vi "VISCOSITY.vi"(0 "SPIN (F)":bool, 1 "Zero? (T)":bool=TRUE, 3 "Startup RPM":dbl=6.0, 5 "LogData? (T)":bool=TRUE, 9 "GUID":string, 11 "DataPoints":i32=10, 12 "stabilization (ms)":u32=10000) -> (4 "cP_Array":dbl[](array[numeric]), 6 "TorqueArray":dbl[](array[numeric]), 8 "final_RPM":dbl, 10 "cP_mean":dbl format="%0.2f", 13 "tau_std":dbl format="%0.2f", 14 "ET (s)":dbl, 15 "tau_mean":dbl format="%0.2f")   [LabVIEW 2019]
uses:
  CurrentRevision/5_Controls/Brookfield_type-def.ctl
  <vilib>/Instr/_visa.llb/VISA Flush IO Buffer Mask.ctl
  <vilib>/Utility/error.llb/DialogType.ctl
  <vilib>/Analysis/baseanly.llb/Mean (DBL).vi
  <vilib>/Utility/file.llb/Read Delimited Spreadsheet (DBL).vi
  <vilib>/Analysis/NI_AALBase.lvlib
panel:
  out "READ_COUNT_AT_SPEED":i32
  out "end_time":timestamp
  out "start_time":timestamp
  out "Temp_mean":dbl format="%0.2f"
  out "Coefficient of VariationT":dbl
  out "net tq%":dbl
  out "Desired RPM":dbl
  out "Coefficient of Variation cP":dbl
  out "speed ratio":dbl
  out "cP":dbl
  out "Loop Tracker":T1[](array[typedef])
  out "Zero_write":dbl
  out "Set RPM":dbl
  out "standard dev":dbl format="%0.2f"
  out "Zero_read":dbl
  out "ReconnectAttempts":i32
  out "log_string":string
  out "TempArray":dbl[](array[numeric])
  out "error out":errorcluster
  out "Enum":T1
  out "temp":dbl
  out "abs tq%":dbl
  out "Control Circuitry Enabled":bool
  out "Motor On":bool
  out "Motor Stopped":bool
  out "Auto-zero Complete":bool
  out "Motor Circuit Error":bool
  out "Diagnostics Error":bool
  out "Invalid Command Received":bool
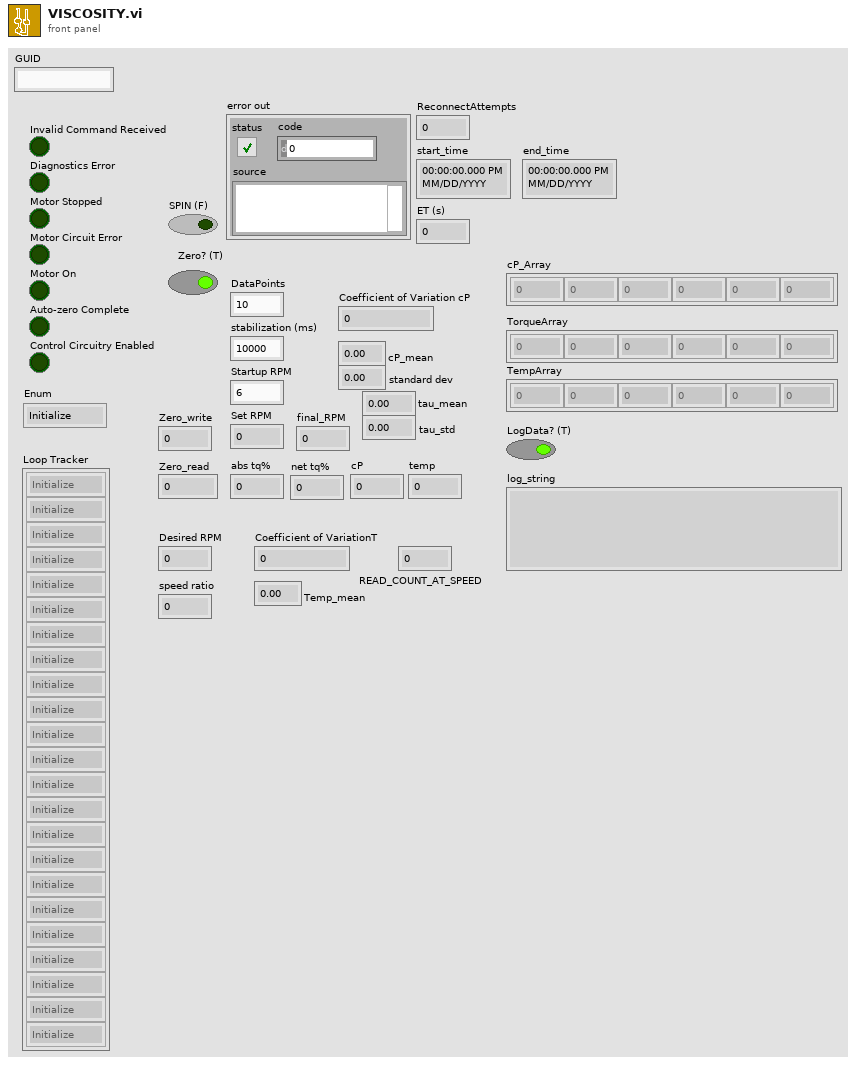
[diagram p1: front panel]
types:
  T1 = typedef "Brookfield_type-def.ctl" = enum16{"Initialize", "Enable", "Ready", "Zero", "Set Speed", "Read", "Stop Motor", "Error", "Disconnect"}
  T2 = enum16{"open", "replace", "create", "open or create", "replace or create", "replace or create with confirmation"}
  T3 = typedef "VISA Flush IO Buffer Mask.ctl" = u16
  T4 = typedef "DialogType.ctl" = u16
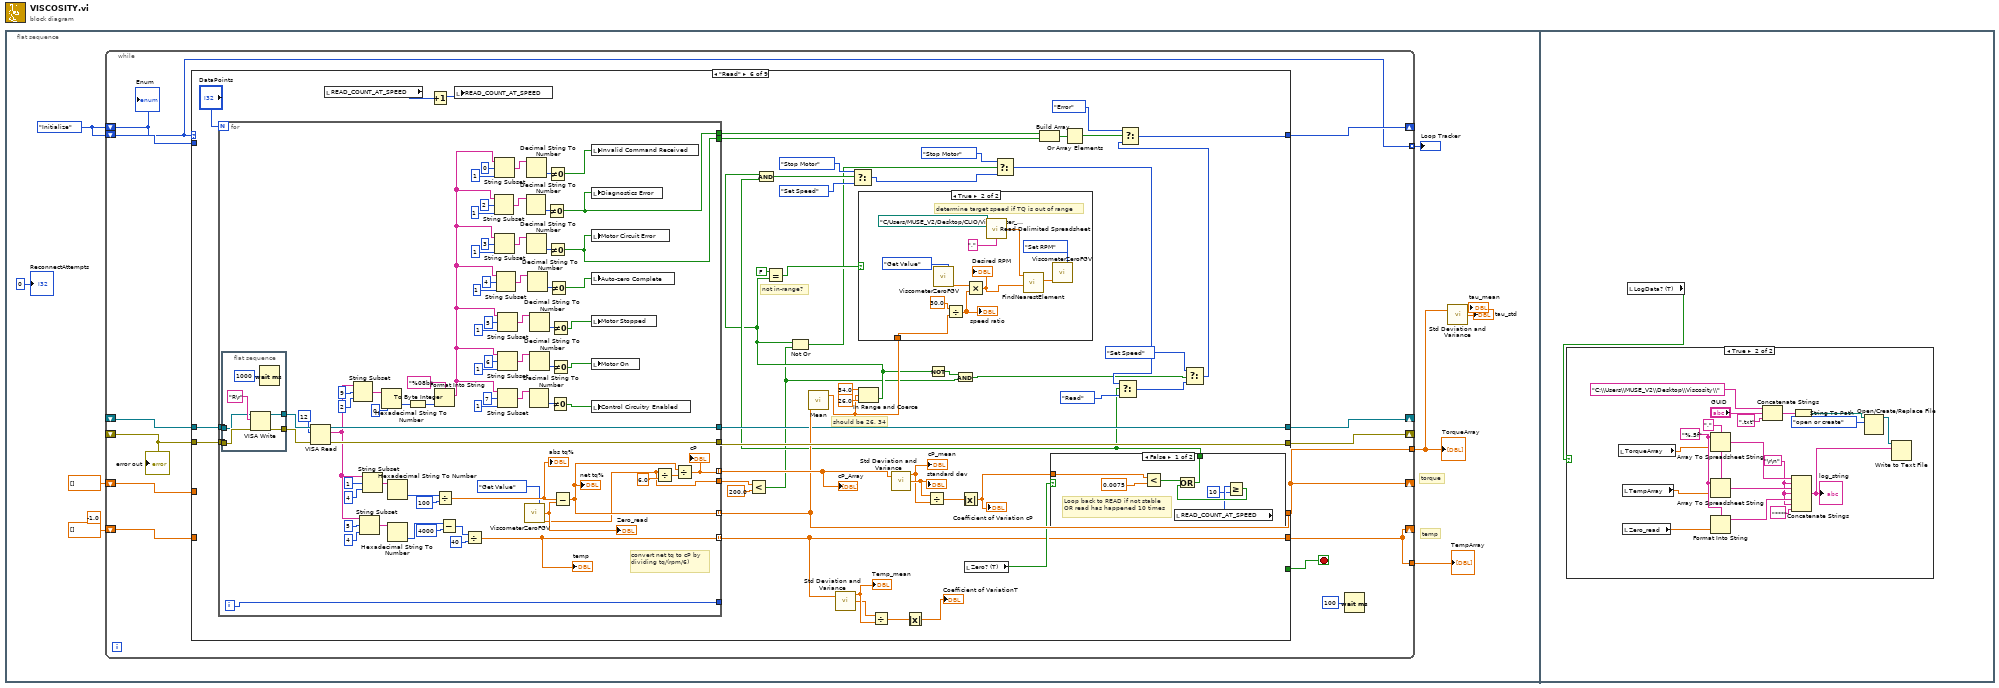
[diagram p0: block diagram]
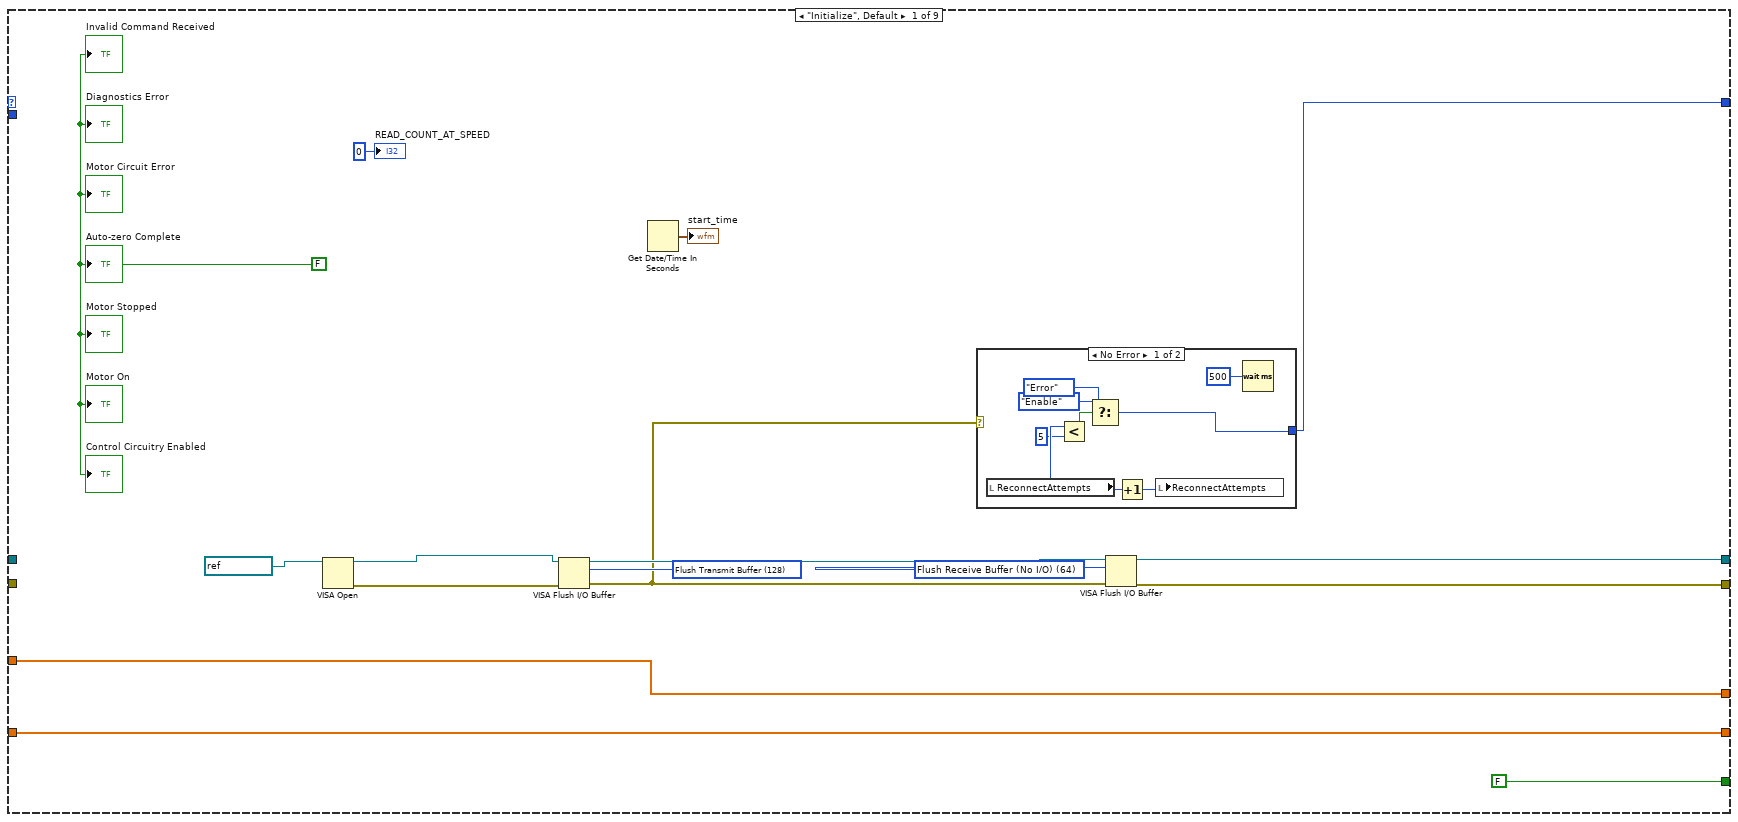
[diagram p2: hidden frame]
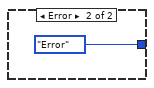
[diagram p3: hidden frame]
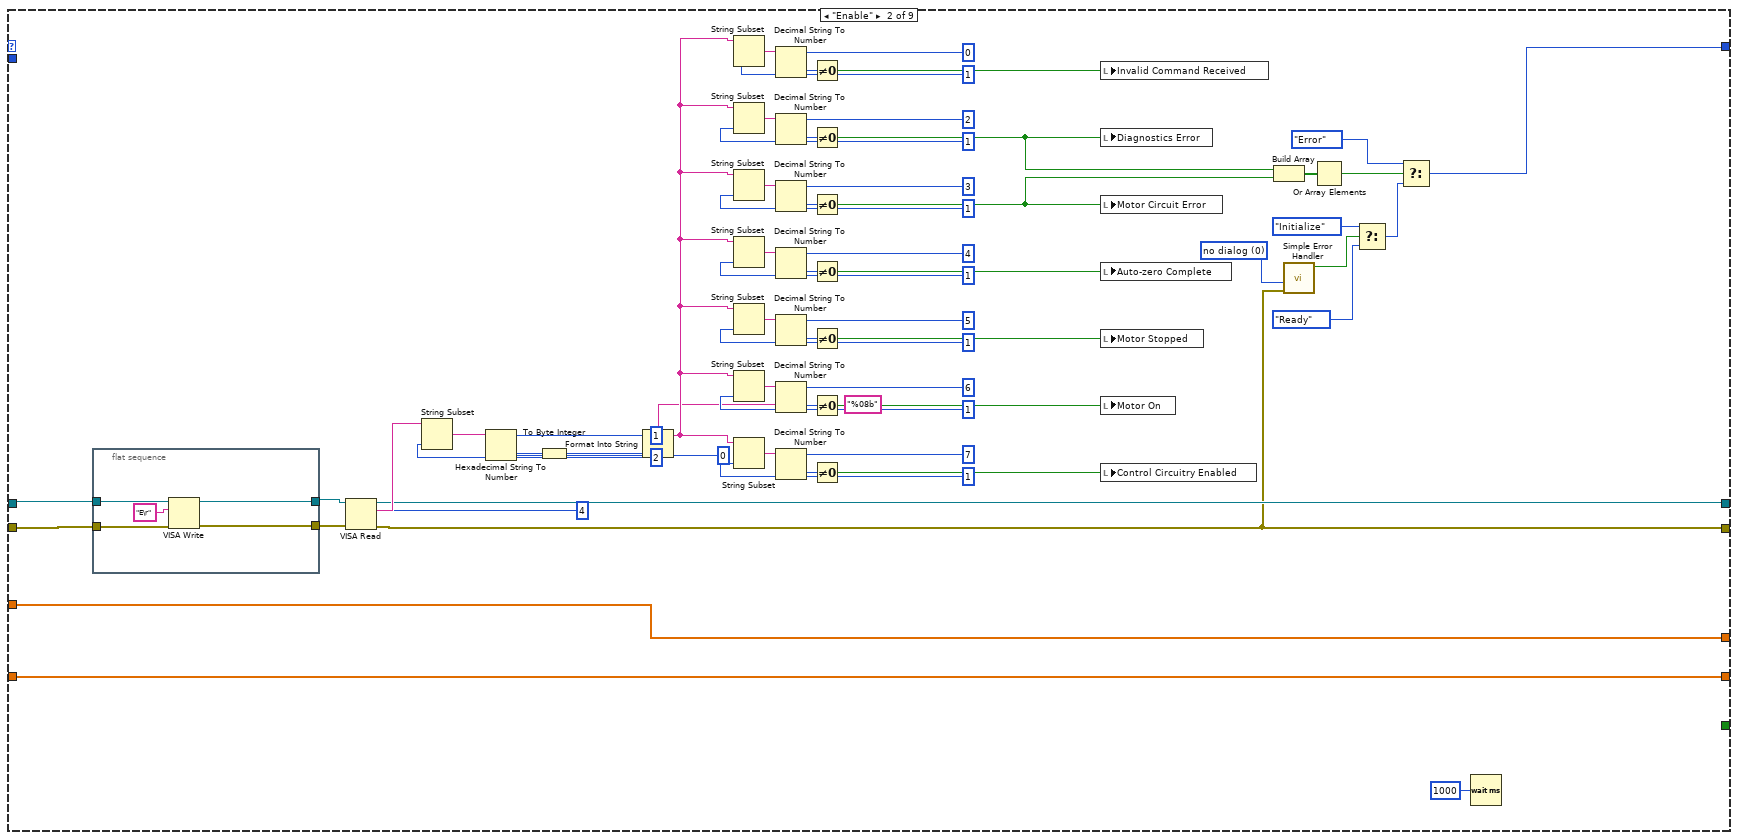
[diagram p4: hidden frame]
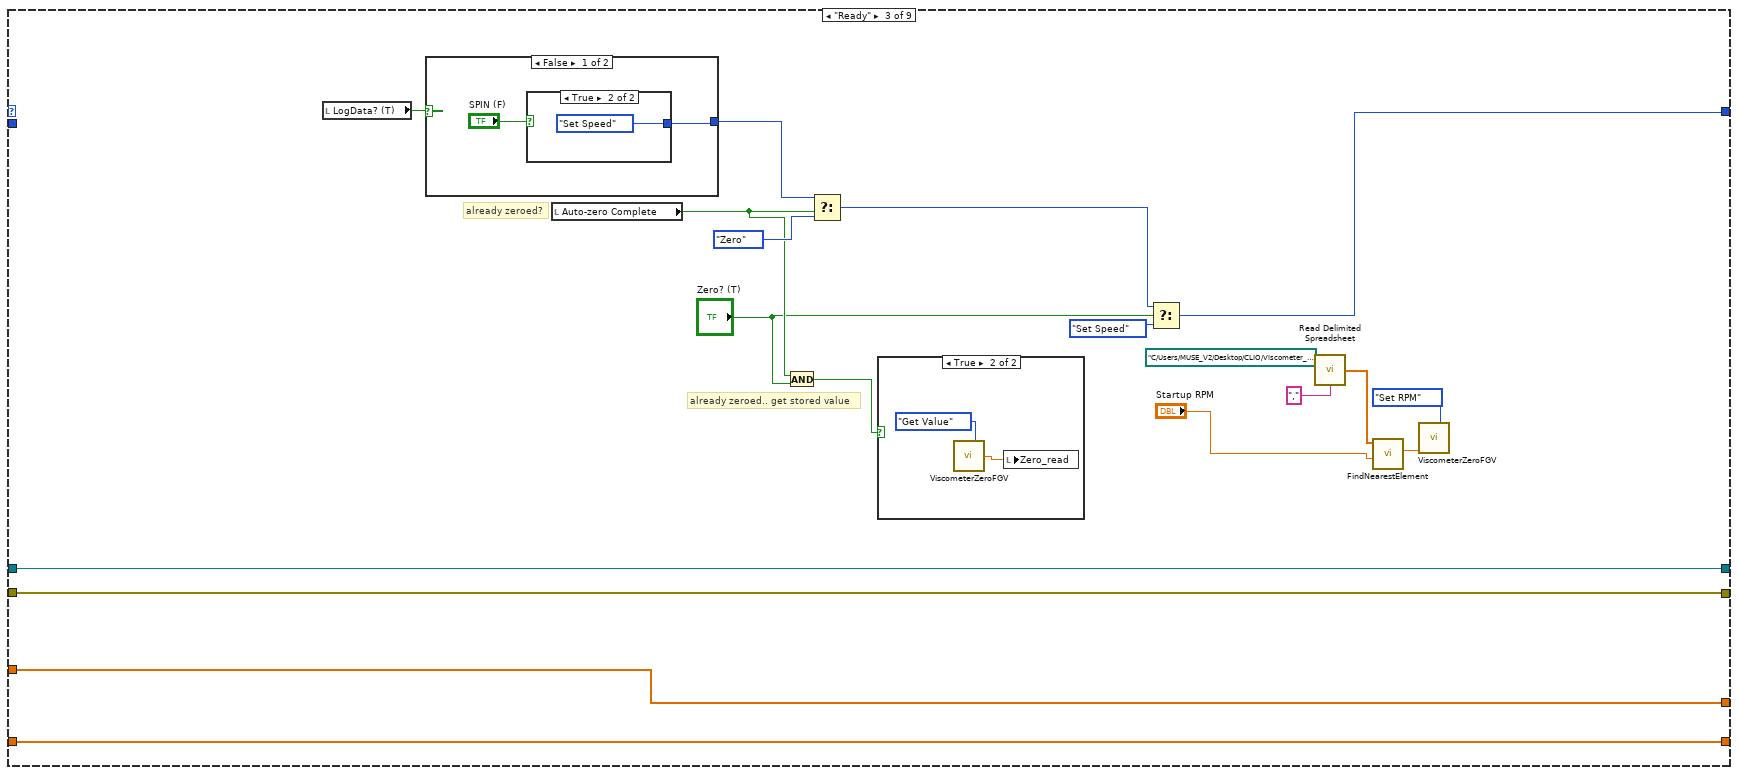
[diagram p5: hidden frame]
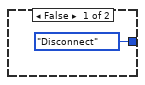
[diagram p6: hidden frame]
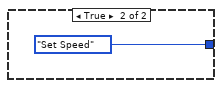
[diagram p7: hidden frame]
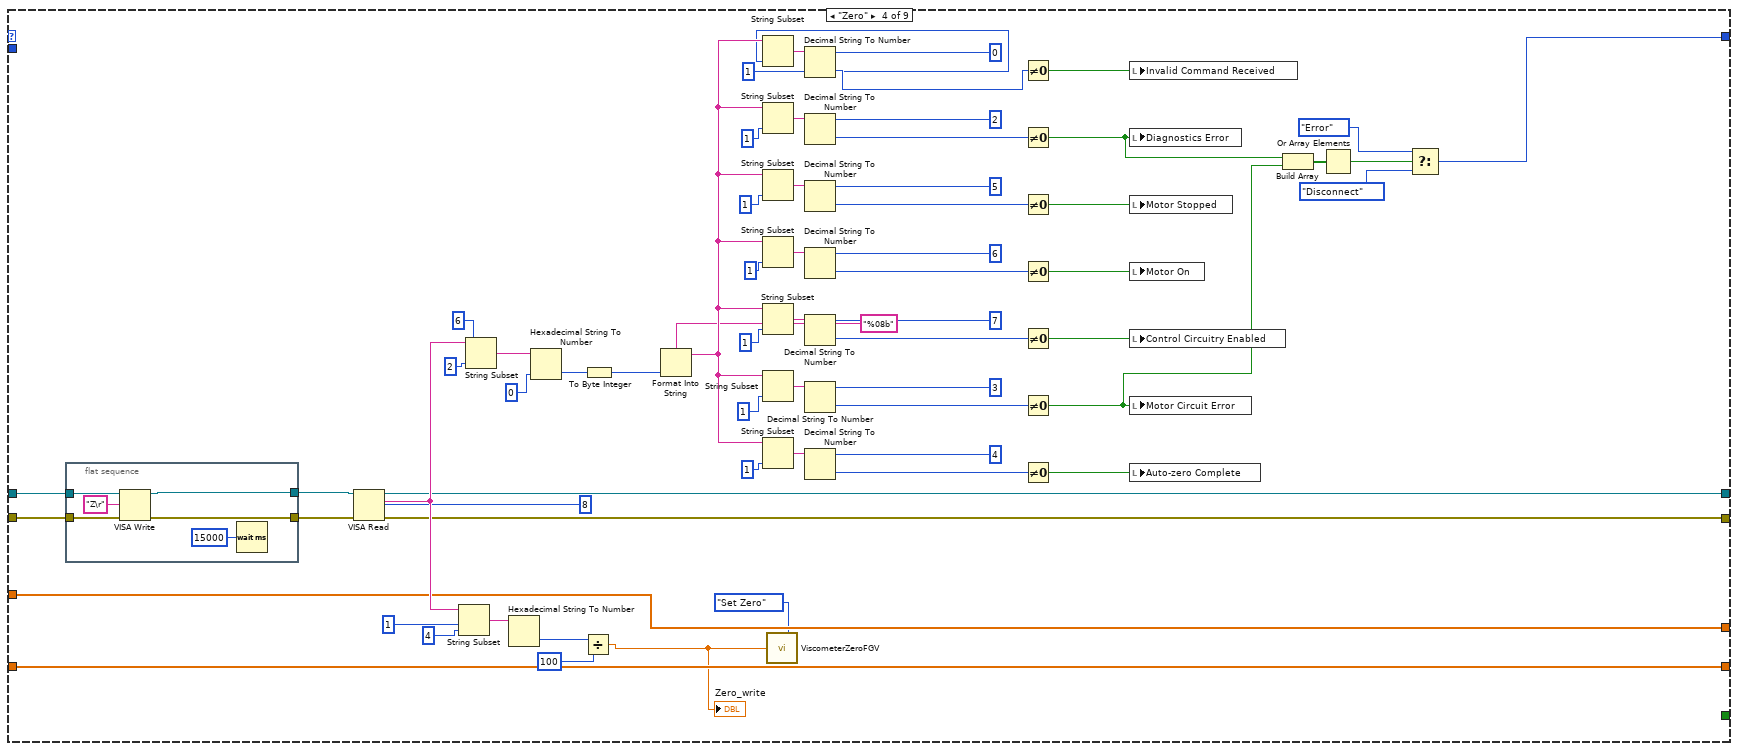
[diagram p9: hidden frame]
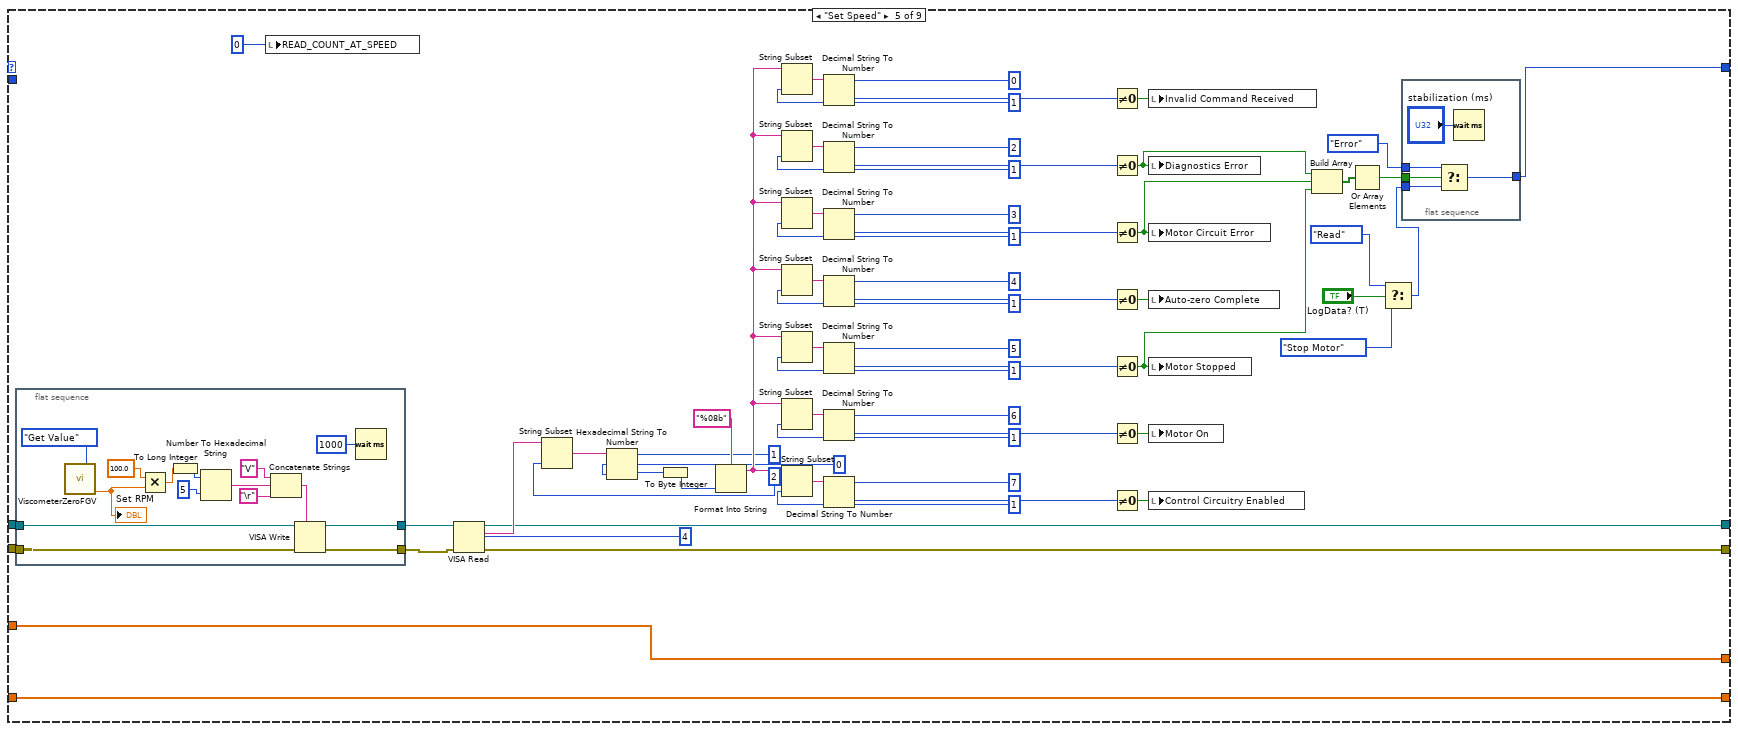
[diagram p10: hidden frame]
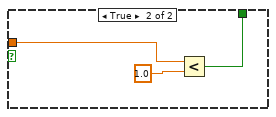
[diagram p11: hidden frame]
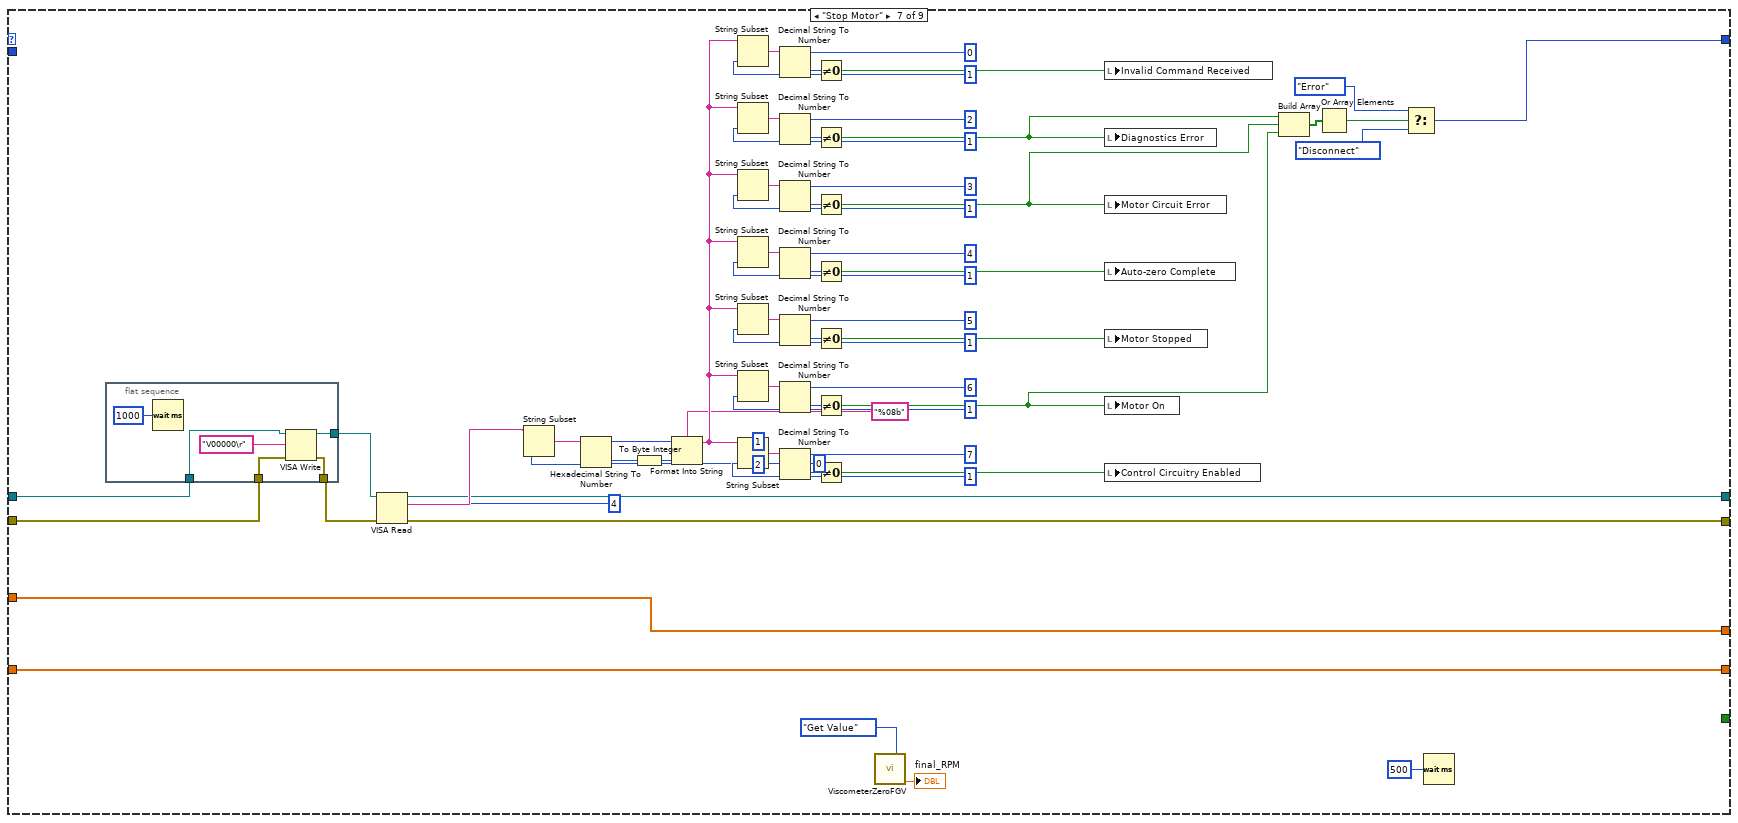
[diagram p13: hidden frame]
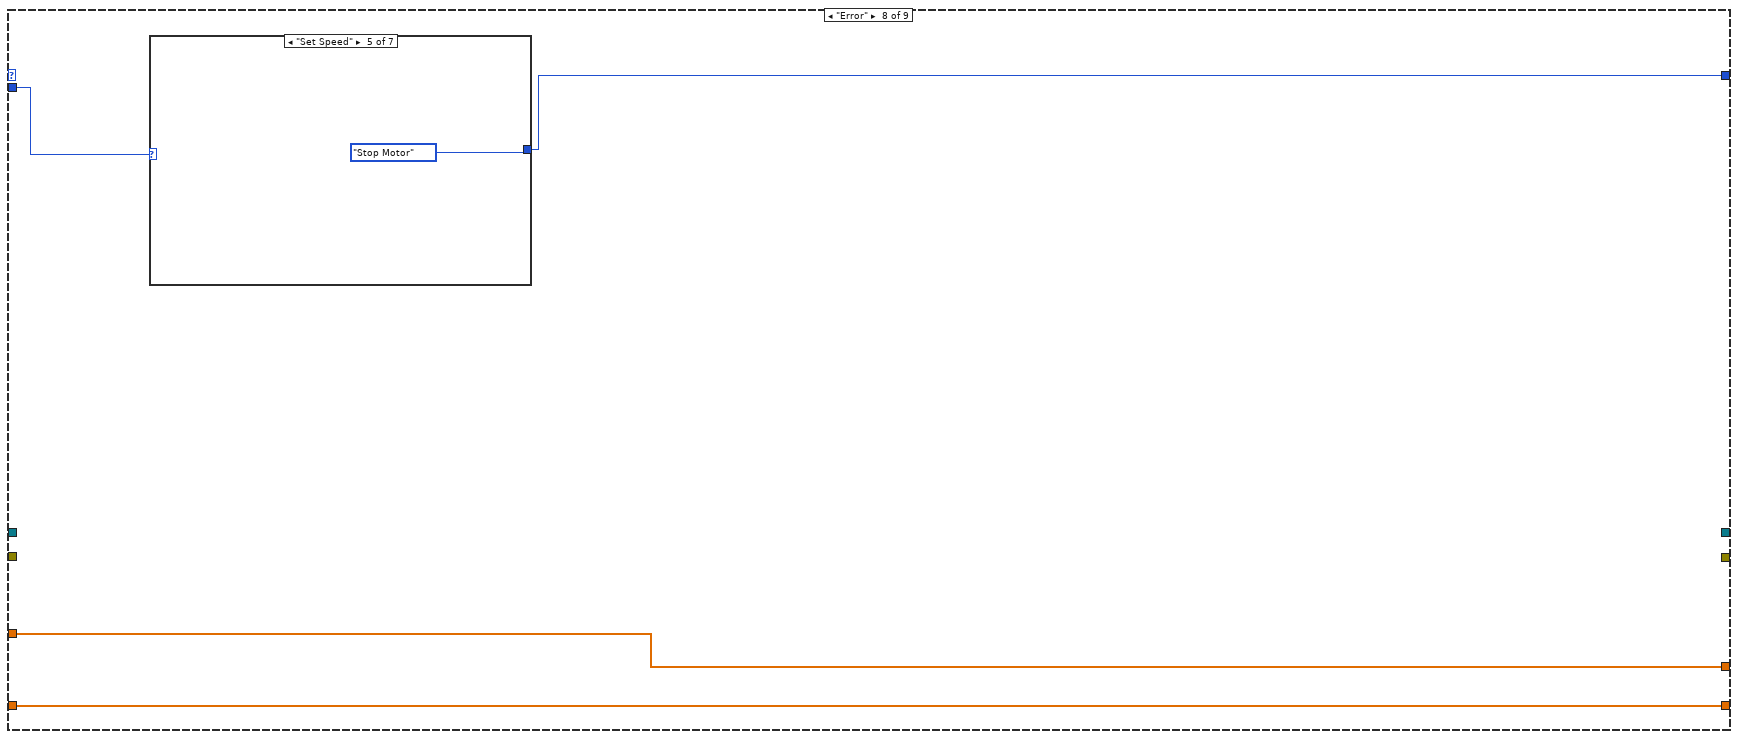
[diagram p14: hidden frame]
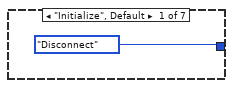
[diagram p15: hidden frame]
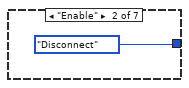
[diagram p16: hidden frame]
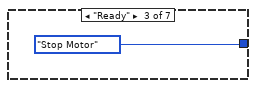
[diagram p17: hidden frame]
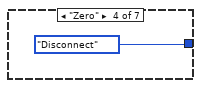
[diagram p18: hidden frame]
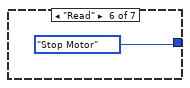
[diagram p19: hidden frame]
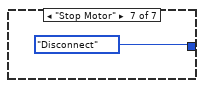
[diagram p20: hidden frame]
diagram:
  n1 = flat-sequence {
    frame #0 {
      (unwired) -1.0
      w9 = Brookfield_type-def."Initialize"
      # "temp"
      # "torque"
      n2 = while {
        shift-right: [w11] -> _
        shift-left: w9 -> [w10]
        shift-right: [w22] -> _
        shift-left: _ -> [w20]
        shift-right: [w21] -> _
        shift-left: _ -> [w19]
        shift-right: [w13] -> _
        shift-left: dbl[] [] -> [w16]
        shift-right: [w12] -> _
        shift-left: dbl[] [] -> [w15]
        shift-left: w9 -> [w17]
        tunnel: [w13] -> w3
        tunnel: [w12] -> w6
        tunnel: [w10] -> w4 mode=indexing
        stop <- w18 stop-if-true
        n3 = case shown="\"Read\"" w10 {
          tunnel: [w26 w65 w131 w153 w232 w318 w460 _ _] -> w22
          tunnel: [w25 w49 w132 w154 w233 w342 w461 _ _] -> w21
          tunnel: w20 -> [_ w110 w131 w156 w220 w334 w448 _ w525]
          tunnel: w19 -> [_ w109 w132 w155 w221 w335 w449 _ w524]
          tunnel: [FALSE _ _ _ _ _ _ _ w523] -> w18
          tunnel: [w35 w59 w129 w146 w228 w338 w455 w513 _] -> w11
          tunnel: [w34 w58 w134 w145 w223 w324 w451 w512 w522] -> w13
          tunnel: [w33 w57 w133 w144 w222 w306 w450 w511 w521] -> w12
          tunnel: w17 -> [_ _ _ _ _ _ _ w510 _]
          tunnel: w16 -> [w34 w58 w134 w145 w223 _ w451 w512 w522]
          tunnel: w15 -> [w33 w57 w133 w144 w222 _ w450 w511 w521]
          frame "Initialize", Default {
            w27 = T3 64 items=["Flush Receive Buffer"=16, "Write Transmit Buffer to Device"=32, "Flush Receive Buffer (No I/O)"=64, "Flush Transmit Buffer"=128] ("Mask")
            w30 = T3 128 items=["Flush Receive Buffer"=16, "Write Transmit Buffer to Device"=32, "Flush Receive Buffer (No I/O)"=64, "Flush Transmit Buffer"=128] ("Mask")
            w37 = FALSE
            n4 = VISA Open(VISA resource name=refnum<visa-resource-name> "COM10" ("Conductivity Port")) -> (VISA resource name=w31:refnum<visa-resource-name>, error out=w32:errorcluster)  [unwired: 4 in]
            n5 = VISA Flush I/O Buffer(VISA resource name=w31, mask (16)=w30, error in (no error)=w32) -> (VISA resource name out=w29:refnum<visa-resource-name>, error out=w28:errorcluster)
            n6 = Get Date/Time In Seconds() -> (seconds since 1Jan1904=→"start_time":timestamp)
            n7 = case shown="No Error" w28 {
              tunnel: [w41 Brookfield_type-def."Error"] -> w35
              frame No Error {
                n8 = local read "ReconnectAttempts"() -> (w44:i32)
                n9 = Less?(x=w44, y=5) -> (x < y?=w42:bool)
                n10 = Select(t=Brookfield_type-def."Enable", s=w42, f=Brookfield_type-def."Error") -> (s? t:f=w41:T1)
                n11 = Increment(x=w44) -> (x+1=w45:i32)
                n12 = local write "ReconnectAttempts"(w45) -> ()
                n13 = Wait (ms)(milliseconds to wait=u32 500) -> ()  [unwired: 1 out]
              }
              frame Error {
              }
            }
            n14 = VISA Flush I/O Buffer(VISA resource name=w29, mask (16)=w27, error in (no error)=w28) -> (VISA resource name out=w26:refnum<visa-resource-name>, error out=w25:errorcluster)
            "Invalid Command Received" <- w37
            "Diagnostics Error" <- w37
            "Motor Circuit Error" <- w37
            "Auto-zero Complete" <- w37
            "Motor Stopped" <- w37
            "Motor On" <- w37
            "Control Circuitry Enabled" <- w37
            "READ_COUNT_AT_SPEED" <- 0
          }
          frame "Enable" {
            w51 = T4 0 items=["no dialog", "OK message", "continue or stop message", "OK message + warnings", "continue/stop + warnings"] ("type of dialog (OK msg:1)")
            n15 = flat-sequence {
              tunnel: w110 -> [w114]
              tunnel: w109 -> [w113]
              tunnel: [w112] -> w50
              tunnel: [w111] -> w66
              frame #0 {
                n16 = VISA Write(VISA resource name=w114, write buffer="E\r", error in (no error)=w113) -> (VISA resource name out=w111:refnum<visa-resource-name>, error out=w112:errorcluster)  [unwired: 1 out]
              }
            }
            n17 = VISA Read(VISA resource name=w66, byte count=u32 4, error in (no error)=w50) -> (VISA resource name out=w65:refnum<visa-resource-name>, read buffer=w108:string, error out=w49:errorcluster)  [unwired: 1 out]
            n18 = String Subset(string=w108, offset (0)=1, length (rest)=2 ("length (rest)")) -> (substring=w102:string)
            n19 = Hexadecimal String To Number(string=w102, default (0uL)=u32 0 ("default (0 U32)")) -> (number=w98:u32)  [unwired: 1 in, 1 out]
            n20 = To Byte Integer(number=w98) -> (8bit integer=w99:i8)
            n21 = Format Into String(format string="%08b", w99) -> (resulting string=w85:string)  [unwired: 2 in, 1 out]
            n22 = String Subset(string=w85, offset (0)=0, length (rest)=1 ("length (rest)")) -> (substring=w101:string)
            n23 = String Subset(string=w85, offset (0)=2, length (rest)=1 ("length (rest)")) -> (substring=w96:string)
            n24 = String Subset(string=w85, offset (0)=3, length (rest)=1 ("length (rest)")) -> (substring=w95:string)
            n25 = String Subset(string=w85, offset (0)=4, length (rest)=1 ("length (rest)")) -> (substring=w92:string)
            n26 = String Subset(string=w85, offset (0)=5, length (rest)=1 ("length (rest)")) -> (substring=w91:string)
            n27 = String Subset(string=w85, offset (0)=6, length (rest)=1 ("length (rest)")) -> (substring=w88:string)
            n28 = String Subset(string=w85, offset (0)=7, length (rest)=1 ("length (rest)")) -> (substring=w87:string)
            n29 = Decimal String To Number(string=w101) -> (number=w100:i32)  [unwired: 2 in, 1 out]
            n30 = Decimal String To Number(string=w96) -> (number=w97:i32)  [unwired: 2 in, 1 out]
            n31 = Decimal String To Number(string=w95) -> (number=w94:i32)  [unwired: 2 in, 1 out]
            n32 = Decimal String To Number(string=w92) -> (number=w93:i32)  [unwired: 2 in, 1 out]
            n33 = Decimal String To Number(string=w91) -> (number=w90:i32)  [unwired: 2 in, 1 out]
            n34 = Decimal String To Number(string=w88) -> (number=w89:i32)  [unwired: 2 in, 1 out]
            n35 = Decimal String To Number(string=w87) -> (number=w86:i32)  [unwired: 2 in, 1 out]
            n36 = Not Equal To 0?(x=w100) -> (x != 0?=w103:bool)
            n37 = Not Equal To 0?(x=w97) -> (x != 0?=w64:bool)
            n38 = Not Equal To 0?(x=w94) -> (x != 0?=w63:bool)
            n39 = Not Equal To 0?(x=w93) -> (x != 0?=w104:bool)
            n40 = Not Equal To 0?(x=w90) -> (x != 0?=w105:bool)
            n41 = Not Equal To 0?(x=w89) -> (x != 0?=w106:bool)
            n42 = Not Equal To 0?(x=w86) -> (x != 0?=w107:bool)
            n43 = local write "Invalid Command Received"(w103) -> ()
            n44 = local write "Diagnostics Error"(w64) -> ()
            n45 = local write "Motor Circuit Error"(w63) -> ()
            n46 = local write "Auto-zero Complete"(w104) -> ()
            n47 = local write "Motor Stopped"(w105) -> ()
            n48 = local write "Motor On"(w106) -> ()
            n49 = local write "Control Circuitry Enabled"(w107) -> ()
            n50 = Build Array(w64, w63) -> (w62:bool[])
            n51 = call <vilib>:"Simple Error Handler.vi"("type of dialog (OK msg:1)"=w51, "error in (no error)"=w49) -> ("error?"=w53:bool)  [unwired: 3 in, 4 out]
            n52 = Or Array Elements(Boolean array=w62) -> (logical OR=w61:bool)
            n53 = Select(t=Brookfield_type-def."Initialize", s=w53, f=Brookfield_type-def."Ready") -> (s? t:f=w56:T1)
            n54 = Select(t=Brookfield_type-def."Error", s=w61, f=w56) -> (s? t:f=w59:T1)
            n55 = Wait (ms)(milliseconds to wait=u32 1000) -> ()  [unwired: 1 out]
          }
          frame "Ready" {
            # "already zeroed?"
            # "already zeroed.. get stored value"
            n56 = local read "LogData? (T)"() -> (w122:bool)
            n57 = case shown="False" w122 {
              tunnel: [w136 Brookfield_type-def."Set Speed" ("t")] -> w126
              frame False {
                n58 = case shown="True" "SPIN (F)" {
                  tunnel: [Brookfield_type-def."Disconnect" ("t") Brookfield_type-def."Set Speed" ("t")] -> w136
                  frame False {
                  }
                  frame True {
                  }
                }
              }
              frame True {
              }
            }
            n59 = local read "Auto-zero Complete"() -> (w125:bool)
            n60 = And(x=w125, y="Zero? (T)") -> (x .and. y?=w123:bool)
            n61 = Select(t=w126, s=w125, f=Brookfield_type-def."Zero") -> (s? t:f=w128:T1)
            n62 = case shown="True" w123 {
              frame False {
              }
              frame True {
                n63 = call "ViscometerZeroFGV.vi"("Enum"=enum16{"Set RPM", "Set Zero", "Get Value"}."Get Value") -> ("Zero_read"=w140:dbl)  [unwired: 13 in, 1 out]
                n64 = local write "Zero_read"(w140) -> ()
              }
            }
            n65 = Select(t=w128, s="Zero? (T)", f=Brookfield_type-def."Set Speed") -> (s? t:f=w129:T1)
            n66 = call-poly <vilib>:"Read Delimited Spreadsheet.vi"("file path (dialog if empty)"=path "C:/Users/MUSE_V2/Desktop/CLIO/Viscometer_Speed_Sets.csv", "delimiter (\\t)"="," ("delimiter (\\t)")) -> ("first row"=w119:dbl[])  [unwired: 8 in, 5 out]
            n67 = call "FindNearestElement.vi"("Desired Element"="Startup RPM", "Input Array"=w119) -> ("Closest Element"=w121:dbl)  [unwired: 8 in, 1 out]
            n68 = call "ViscometerZeroFGV.vi"("Enum"=enum16{"Set RPM", "Set Zero", "Get Value"}."Set RPM", "RPM_write"=w121) -> ()  [unwired: 12 in, 2 out]
          }
          frame "Zero" {
            n69 = flat-sequence {
              tunnel: [w212] -> w180
              tunnel: [w211] -> w179
              tunnel: w156 -> [w209]
              tunnel: w155 -> [w208]
              frame #0 {
                n70 = VISA Write(VISA resource name=w209, write buffer="Z\r", error in (no error)=w208) -> (VISA resource name out=w211:refnum<visa-resource-name>, error out=w212:errorcluster)  [unwired: 1 out]
                n71 = Wait (ms)(milliseconds to wait=u32 15000) -> ()  [unwired: 1 out]
              }
            }
            n72 = VISA Read(VISA resource name=w179, byte count=u32 8, error in (no error)=w180) -> (VISA resource name out=w153:refnum<visa-resource-name>, read buffer=w201:string, error out=w154:errorcluster)  [unwired: 1 out]
            n73 = String Subset(string=w201, offset (0)=1, length (rest)=4 ("length (rest)")) -> (substring=w181:string)
            n74 = String Subset(string=w201, offset (0)=6, length (rest)=2 ("length (rest)")) -> (substring=w183:string)
            n75 = Hexadecimal String To Number(string=w181) -> (number=w182:u32)  [unwired: 2 in, 1 out]
            n76 = Hexadecimal String To Number(string=w183, default (0uL)=u32 0 ("default (0 U32)")) -> (number=w187:u32)  [unwired: 1 in, 1 out]
            n77 = Divide(x=w182, y=u32 100) -> (x/y=w143:dbl)
            "Zero_write" <- w143
            n78 = To Byte Integer(number=w187) -> (8bit integer=w186:i8)
            n79 = Format Into String(format string="%08b", w186) -> (resulting string=w200:string)  [unwired: 2 in, 1 out]
            n80 = String Subset(string=w200, offset (0)=0, length (rest)=1 ("length (rest)")) -> (substring=w184:string)
            n81 = String Subset(string=w200, offset (0)=2, length (rest)=1 ("length (rest)")) -> (substring=w189:string)
            n82 = String Subset(string=w200, offset (0)=5, length (rest)=1 ("length (rest)")) -> (substring=w194:string)
            n83 = String Subset(string=w200, offset (0)=6, length (rest)=1 ("length (rest)")) -> (substring=w197:string)
            n84 = String Subset(string=w200, offset (0)=7, length (rest)=1 ("length (rest)")) -> (substring=w198:string)
            n85 = String Subset(string=w200, offset (0)=3, length (rest)=1 ("length (rest)")) -> (substring=w190:string)
            n86 = String Subset(string=w200, offset (0)=4, length (rest)=1 ("length (rest)")) -> (substring=w193:string)
            n87 = call "ViscometerZeroFGV.vi"("Enum"=enum16{"Set RPM", "Set Zero", "Get Value"}."Set Zero", "Zero_write"=w143) -> ()  [unwired: 12 in, 2 out]
            n88 = Decimal String To Number(string=w184) -> (number=w185:i32)  [unwired: 2 in, 1 out]
            n89 = Decimal String To Number(string=w189) -> (number=w188:i32)  [unwired: 2 in, 1 out]
            n90 = Decimal String To Number(string=w194) -> (number=w195:i32)  [unwired: 2 in, 1 out]
            n91 = Decimal String To Number(string=w197) -> (number=w196:i32)  [unwired: 2 in, 1 out]
            n92 = Decimal String To Number(string=w198) -> (number=w199:i32)  [unwired: 2 in, 1 out]
            n93 = Decimal String To Number(string=w190) -> (number=w191:i32)  [unwired: 2 in, 1 out]
            n94 = Decimal String To Number(string=w193) -> (number=w192:i32)  [unwired: 2 in, 1 out]
            n95 = Not Equal To 0?(x=w185) -> (x != 0?=w206:bool)
            n96 = Not Equal To 0?(x=w188) -> (x != 0?=w148:bool)
            n97 = Not Equal To 0?(x=w195) -> (x != 0?=w204:bool)
            n98 = Not Equal To 0?(x=w196) -> (x != 0?=w203:bool)
            n99 = Not Equal To 0?(x=w199) -> (x != 0?=w202:bool)
            n100 = Not Equal To 0?(x=w191) -> (x != 0?=w147:bool)
            n101 = Not Equal To 0?(x=w192) -> (x != 0?=w205:bool)
            n102 = local write "Invalid Command Received"(w206) -> ()
            n103 = local write "Diagnostics Error"(w148) -> ()
            n104 = local write "Motor Stopped"(w204) -> ()
            n105 = local write "Motor On"(w203) -> ()
            n106 = local write "Control Circuitry Enabled"(w202) -> ()
            n107 = local write "Motor Circuit Error"(w147) -> ()
            n108 = local write "Auto-zero Complete"(w205) -> ()
            n109 = Build Array(w148, w147) -> (w152:bool[])
            n110 = Or Array Elements(Boolean array=w152) -> (logical OR=w151:bool)
            n111 = Select(t=Brookfield_type-def."Error", s=w151, f=Brookfield_type-def."Disconnect") -> (s? t:f=w146:T1)
          }
          frame "Set Speed" {
            n112 = flat-sequence {
              tunnel: w221 -> [w287]
              tunnel: w220 -> [w286]
              tunnel: [w285] -> w219
              tunnel: [w284] -> w218
              frame #0 {
                n113 = call "ViscometerZeroFGV.vi"("Enum"=enum16{"Set RPM", "Set Zero", "Get Value"}."Get Value") -> ("RPM_read"=w281:dbl)  [unwired: 13 in, 1 out]
                "Set RPM" <- w281
                n114 = Multiply(x=100.0, y=w281) -> (x*y=w283:dbl)
                n115 = To Long Integer(number=w283) -> (32bit integer=w282:i32)
                n116 = Number To Hexadecimal String(1:i16 5 ("width (-)"), 2:w282) -> (0:w293:string)
                n117 = Concatenate Strings("V" ("string"), w293, "\r") -> (w292:string)
                n118 = VISA Write(VISA resource name=w286, write buffer=w292, error in (no error)=w287) -> (VISA resource name out=w284:refnum<visa-resource-name>, error out=w285:errorcluster)  [unwired: 1 out]
                n119 = Wait (ms)(milliseconds to wait=u32 1000) -> ()  [unwired: 1 out]
              }
            }
            n120 = local write "READ_COUNT_AT_SPEED"(0) -> ()
            n121 = VISA Read(VISA resource name=w218, byte count=u32 4, error in (no error)=w219) -> (VISA resource name out=w232:refnum<visa-resource-name>, read buffer=w274:string, error out=w233:errorcluster)  [unwired: 1 out]
            n122 = String Subset(string=w274, offset (0)=1, length (rest)=2 ("length (rest)")) -> (substring=w270:string)
            n123 = Hexadecimal String To Number(string=w270, default (0uL)=u32 0 ("default (0 U32)")) -> (number=w266:u32)  [unwired: 1 in, 1 out]
            n124 = To Byte Integer(number=w266) -> (8bit integer=w267:i8)
            n125 = Format Into String(format string="%08b", w267) -> (resulting string=w253:string)  [unwired: 2 in, 1 out]
            n126 = String Subset(string=w253, offset (0)=0, length (rest)=1 ("length (rest)")) -> (substring=w269:string)
            n127 = String Subset(string=w253, offset (0)=2, length (rest)=1 ("length (rest)")) -> (substring=w264:string)
            n128 = String Subset(string=w253, offset (0)=3, length (rest)=1 ("length (rest)")) -> (substring=w263:string)
            n129 = String Subset(string=w253, offset (0)=4, length (rest)=1 ("length (rest)")) -> (substring=w260:string)
            n130 = String Subset(string=w253, offset (0)=5, length (rest)=1 ("length (rest)")) -> (substring=w259:string)
            n131 = String Subset(string=w253, offset (0)=6, length (rest)=1 ("length (rest)")) -> (substring=w256:string)
            n132 = String Subset(string=w253, offset (0)=7, length (rest)=1 ("length (rest)")) -> (substring=w255:string)
            n133 = Decimal String To Number(string=w269) -> (number=w268:i32)  [unwired: 2 in, 1 out]
            n134 = Decimal String To Number(string=w264) -> (number=w265:i32)  [unwired: 2 in, 1 out]
            n135 = Decimal String To Number(string=w263) -> (number=w262:i32)  [unwired: 2 in, 1 out]
            n136 = Decimal String To Number(string=w260) -> (number=w261:i32)  [unwired: 2 in, 1 out]
            n137 = Decimal String To Number(string=w259) -> (number=w258:i32)  [unwired: 2 in, 1 out]
            n138 = Decimal String To Number(string=w256) -> (number=w257:i32)  [unwired: 2 in, 1 out]
            n139 = Decimal String To Number(string=w255) -> (number=w254:i32)  [unwired: 2 in, 1 out]
            n140 = Not Equal To 0?(x=w268) -> (x != 0?=w271:bool)
            n141 = Not Equal To 0?(x=w265) -> (x != 0?=w226:bool)
            n142 = Not Equal To 0?(x=w262) -> (x != 0?=w227:bool)
            n143 = Not Equal To 0?(x=w261) -> (x != 0?=w272:bool)
            n144 = Not Equal To 0?(x=w258) -> (x != 0?=w224:bool)
            n145 = Not Equal To 0?(x=w257) -> (x != 0?=w225:bool)
            n146 = Not Equal To 0?(x=w254) -> (x != 0?=w273:bool)
            n147 = local write "Invalid Command Received"(w271) -> ()
            n148 = local write "Diagnostics Error"(w226) -> ()
            n149 = local write "Motor Circuit Error"(w227) -> ()
            n150 = local write "Auto-zero Complete"(w272) -> ()
            n151 = local write "Motor Stopped"(w224) -> ()
            n152 = local write "Motor On"(w225) -> ()
            n153 = local write "Control Circuitry Enabled"(w273) -> ()
            n154 = Build Array(w226, w227, w224) -> (w231:bool[])
            n155 = Or Array Elements(Boolean array=w231) -> (logical OR=w230:bool)
            n156 = Select(t=Brookfield_type-def."Read", s="LogData? (T)", f=Brookfield_type-def."Stop Motor") -> (s? t:f=w215:T1)
            n157 = flat-sequence {
              tunnel: w230 -> [w279]
              tunnel: w215 -> [w278]
              tunnel: Brookfield_type-def."Error" -> [w277]
              tunnel: [w276] -> w228
              frame #0 {
                n158 = Select(t=w277, s=w279, f=w278) -> (s? t:f=w276:T1)
                n159 = Wait (ms)(milliseconds to wait="stabilization (ms)") -> ()  [unwired: 1 out]
              }
            }
          }
          frame "Read" {
            # "should be 26, 34"
            # "not in-range?"
            n160 = for {
              N: "DataPoints" -> [_]
              tunnel: [w436] -> w318
              tunnel: [w435] -> w342
              tunnel: [w434] -> w337
              tunnel: [w433] -> w336
              tunnel: [w432] -> w306 mode=indexing
              tunnel: [w368] -> w324 mode=indexing
              tunnel: w335 -> [w431]
              tunnel: w334 -> [w430]
              tunnel: [w372] -> _
              tunnel: [w367] -> w332 mode=indexing
              tunnel: [w364] -> w320
              i -> [w372]
              # "convert net tq to cP by dividing tq/(rpm/6)"
              n161 = flat-sequence {
                tunnel: w431 -> [w441]
                tunnel: w430 -> [w439]
                tunnel: [w438] -> w429
                tunnel: [w437] -> w428
                frame #0 {
                  n162 = VISA Write(VISA resource name=w439, write buffer="R\r", error in (no error)=w441) -> (VISA resource name out=w437:refnum<visa-resource-name>, error out=w438:errorcluster)  [unwired: 1 out]
                  n163 = Wait (ms)(milliseconds to wait=u32 1000) -> ()  [unwired: 1 out]
                }
              }
              n164 = VISA Read(VISA resource name=w428, byte count=u32 12, error in (no error)=w429) -> (VISA resource name out=w436:refnum<visa-resource-name>, read buffer=w412:string, error out=w435:errorcluster)  [unwired: 1 out]
              n165 = String Subset(string=w412, offset (0)=9, length (rest)=2 ("length (rest)")) -> (substring=w411:string)
              n166 = String Subset(string=w412, offset (0)=5, length (rest)=4 ("length (rest)")) -> (substring=w418:string)
              n167 = String Subset(string=w412, offset (0)=1, length (rest)=4 ("length (rest)")) -> (substring=w424:string)
              n168 = Hexadecimal String To Number(string=w411, default (0uL)=u32 0 ("default (0 U32)")) -> (number=w403:u32)  [unwired: 1 in, 1 out]
              n169 = Hexadecimal String To Number(string=w424) -> (number=w423:u32)  [unwired: 2 in, 1 out]
              n170 = Hexadecimal String To Number(string=w418) -> (number=w417:u32)  [unwired: 2 in, 1 out]
              n171 = To Byte Integer(number=w403) -> (8bit integer=w404:i8)
              n172 = Format Into String(format string="%08b", w404) -> (resulting string=w378:string)  [unwired: 2 in, 1 out]
              n173 = Divide(x=w423, y=u32 100) -> (x/y=w371:dbl)
              "abs tq%" <- w371
              n174 = Subtract(x=w417, y=u32 4000) -> (x-y=w415:u32)
              n175 = Divide(x=w415, y=u32 40) -> (x/y=w432:dbl)
              "temp" <- w432
              n176 = String Subset(string=w378, offset (0)=2, length (rest)=1 ("length (rest)")) -> (substring=w401:string)
              n177 = String Subset(string=w378, offset (0)=0, length (rest)=1 ("length (rest)")) -> (substring=w407:string)
              n178 = String Subset(string=w378, offset (0)=3, length (rest)=1 ("length (rest)")) -> (substring=w396:string)
              n179 = String Subset(string=w378, offset (0)=4, length (rest)=1 ("length (rest)")) -> (substring=w393:string)
              n180 = String Subset(string=w378, offset (0)=7, length (rest)=1 ("length (rest)")) -> (substring=w380:string)
              n181 = String Subset(string=w378, offset (0)=5, length (rest)=1 ("length (rest)")) -> (substring=w388:string)
              n182 = String Subset(string=w378, offset (0)=6, length (rest)=1 ("length (rest)")) -> (substring=w385:string)
              n183 = call "ViscometerZeroFGV.vi"("Enum"=enum16{"Set RPM", "Set Zero", "Get Value"}."Get Value") -> ("Zero_read"=w366:dbl, "RPM_read"=w364:dbl)  [unwired: 13 in]
              "Zero_read" <- w366
              n184 = Decimal String To Number(string=w401) -> (number=w402:i32)  [unwired: 2 in, 1 out]
              n185 = Decimal String To Number(string=w407) -> (number=w406:i32)  [unwired: 2 in, 1 out]
              n186 = Decimal String To Number(string=w396) -> (number=w395:i32)  [unwired: 2 in, 1 out]
              n187 = Decimal String To Number(string=w393) -> (number=w394:i32)  [unwired: 2 in, 1 out]
              n188 = Decimal String To Number(string=w380) -> (number=w379:i32)  [unwired: 2 in, 1 out]
              n189 = Decimal String To Number(string=w388) -> (number=w387:i32)  [unwired: 2 in, 1 out]
              n190 = Decimal String To Number(string=w385) -> (number=w386:i32)  [unwired: 2 in, 1 out]
              n191 = Not Equal To 0?(x=w402) -> (x != 0?=w434:bool)
              n192 = Not Equal To 0?(x=w406) -> (x != 0?=w373:bool)
              n193 = Not Equal To 0?(x=w395) -> (x != 0?=w433:bool)
              n194 = Not Equal To 0?(x=w394) -> (x != 0?=w374:bool)
              n195 = Not Equal To 0?(x=w379) -> (x != 0?=w377:bool)
              n196 = Not Equal To 0?(x=w387) -> (x != 0?=w375:bool)
              n197 = Not Equal To 0?(x=w386) -> (x != 0?=w376:bool)
              n198 = Subtract(x=w371, y=w366) -> (x-y=w368:dbl)
              "net tq%" <- w368
              n199 = local write "Invalid Command Received"(w373) -> ()
              n200 = local write "Diagnostics Error"(w434) -> ()
              n201 = local write "Motor Circuit Error"(w433) -> ()
              n202 = local write "Auto-zero Complete"(w374) -> ()
              n203 = local write "Motor Stopped"(w375) -> ()
              n204 = local write "Motor On"(w376) -> ()
              n205 = local write "Control Circuitry Enabled"(w377) -> ()
              n206 = Divide(x=w364, y=6.0) -> (x/y=w369:dbl)
              n207 = Divide(x=w368, y=w369) -> (x/y=w367:dbl)
              "cP" <- w367
            }
            "cP_Array" <- w332
            n208 = local read "READ_COUNT_AT_SPEED"() -> (w296:i32)
            n209 = Increment(x=w296) -> (x+1=w295:i32)
            n210 = local write "READ_COUNT_AT_SPEED"(w295) -> ()
            n211 = Less?(x=w320, y=200.0) -> (x < y?=w298:bool)
            n212 = call-poly <vilib>:"Mean.vi"("X"=w324) -> ("mean"=w323:dbl)  [unwired: 1 out]
            n213 = call <vilib>:"Std Deviation and Variance.vi"("X"=w306) -> ("mean"=w308:dbl, "standard deviation"=w307:dbl)  [unwired: 1 in, 1 out]
            "Temp_mean" <- w308
            n214 = In Range and Coerce(upper limit=34.0, x=w323, lower limit=26.0) -> (In Range?=w299:bool)  [unwired: 1 out]
            n215 = Equal?(x=FALSE, y=w299) -> (x = y?=w305:bool)
            n216 = Not Or(1:w298, 2:w299) -> (0:w303:bool)
            n217 = case shown="True" w305 {
              tunnel: w323 -> [_ w362]
              frame False {
              }
              frame True {
                # "determine target speed if TQ is out of range"
                n218 = call "ViscometerZeroFGV.vi"("Enum"=enum16{"Set RPM", "Set Zero", "Get Value"}."Get Value") -> ("RPM_read"=w361:dbl)  [unwired: 13 in, 1 out]
                n219 = Divide(x=30.0, y=w362) -> (x/y=w357:dbl)
                "speed ratio" <- w357
                n220 = Multiply(x=w361, y=w357) -> (x*y=w360:dbl)
                "Desired RPM" <- w360
                n221 = call-poly <vilib>:"Read Delimited Spreadsheet.vi"("file path (dialog if empty)"=path "C:/Users/MUSE_V2/Desktop/CLIO/Viscometer_Speed_Sets.csv", "delimiter (\\t)"="," ("delimiter (\\t)")) -> ("first row"=w356:dbl[])  [unwired: 8 in, 5 out]
                n222 = call "FindNearestElement.vi"("Desired Element"=w360, "Input Array"=w356) -> ("Closest Element"=w359:dbl)  [unwired: 8 in, 1 out]
                n223 = call "ViscometerZeroFGV.vi"("Enum"=enum16{"Set RPM", "Set Zero", "Get Value"}."Set RPM", "RPM_write"=w359) -> ()  [unwired: 12 in, 2 out]
              }
            }
            n224 = Divide(x=w307, y=w308) -> (x/y=w309:dbl)
            n225 = call <vilib>:"Std Deviation and Variance.vi"("X"=w332) -> ("mean"=w330:dbl, "standard deviation"=w331:dbl)  [unwired: 1 in, 1 out]
            "cP_mean" <- w330
            "standard dev" <- w331
            n226 = Absolute Value(x=w309) -> (abs(x)=→"Coefficient of VariationT":dbl)
            n227 = Divide(x=w331, y=w330) -> (x/y=w321:dbl)
            n228 = Not(x=w299) -> (.not. x?=w300:bool)
            n229 = And(x=w300, y=w298) -> (x .and. y?=w297:bool)
            n230 = Absolute Value(x=w321) -> (abs(x)=w313:dbl)
            "Coefficient of Variation cP" <- w313
            n231 = local read "Zero? (T)"() -> (w311:bool)
            n232 = Build Array(w337, w336) -> (w339:bool[])
            n233 = case shown="False" w311 {
              tunnel: w313 -> [w348 w351]
              tunnel: [w346 w350] -> w312
              frame False {
                # "Loop back to READ if not stable OR read has happened 10 times"
                n234 = Less?(x=w348, y=0.0075) -> (x < y?=w347:bool)
                n235 = local read "READ_COUNT_AT_SPEED"() -> (w344:i32)
                n236 = Greater Or Equal?(x=w344, y=10) -> (x >= y?=w345:bool)
                n237 = Or(x=w347, y=w345) -> (x .or. y?=w346:bool)
              }
              frame True {
                n238 = Less?(x=w351, y=1.0) -> (x < y?=w350:bool)
              }
            }
            n239 = And(x=w299, y=w312) -> (x .and. y?=w315:bool)
            n240 = Select(t=Brookfield_type-def."Stop Motor" ("f"), s=w315, f=Brookfield_type-def."Set Speed") -> (s? t:f=w316:T1)
            n241 = Select(t=Brookfield_type-def."Stop Motor" ("f"), s=w303, f=w316) -> (s? t:f=w327:T1)
            n242 = Or Array Elements(Boolean array=w339) -> (logical OR=w341:bool)
            n243 = Select(t=w327, s=w312, f=Brookfield_type-def."Read") -> (s? t:f=w302:T1)
            n244 = Select(t=Brookfield_type-def."Set Speed" ("f"), s=w297, f=w302) -> (s? t:f=w304:T1)
            n245 = Select(t=Brookfield_type-def."Error", s=w341, f=w304) -> (s? t:f=w338:T1)
          }
          frame "Stop Motor" {
            n246 = flat-sequence {
              tunnel: w449 -> [w508]
              tunnel: w448 -> [w506]
              tunnel: [w505] -> w447
              tunnel: [w504] -> w446
              frame #0 {
                n247 = Wait (ms)(milliseconds to wait=u32 1000) -> ()  [unwired: 1 out]
                n248 = VISA Write(VISA resource name=w506, write buffer="V00000\r", error in (no error)=w508) -> (VISA resource name out=w504:refnum<visa-resource-name>, error out=w505:errorcluster)  [unwired: 1 out]
              }
            }
            n249 = VISA Read(VISA resource name=w446, byte count=u32 4, error in (no error)=w447) -> (VISA resource name out=w460:refnum<visa-resource-name>, read buffer=w481:string, error out=w461:errorcluster)  [unwired: 1 out]
            n250 = String Subset(string=w481, offset (0)=1, length (rest)=2 ("length (rest)")) -> (substring=w486:string)
            n251 = Hexadecimal String To Number(string=w486, default (0uL)=u32 0 ("default (0 U32)")) -> (number=w490:u32)  [unwired: 1 in, 1 out]
            n252 = To Byte Integer(number=w490) -> (8bit integer=w489:i8)
            n253 = Format Into String(format string="%08b", w489) -> (resulting string=w503:string)  [unwired: 2 in, 1 out]
            n254 = String Subset(string=w503, offset (0)=0, length (rest)=1 ("length (rest)")) -> (substring=w487:string)
            n255 = String Subset(string=w503, offset (0)=2, length (rest)=1 ("length (rest)")) -> (substring=w492:string)
            n256 = String Subset(string=w503, offset (0)=3, length (rest)=1 ("length (rest)")) -> (substring=w493:string)
            n257 = String Subset(string=w503, offset (0)=4, length (rest)=1 ("length (rest)")) -> (substring=w496:string)
            n258 = String Subset(string=w503, offset (0)=5, length (rest)=1 ("length (rest)")) -> (substring=w497:string)
            n259 = String Subset(string=w503, offset (0)=6, length (rest)=1 ("length (rest)")) -> (substring=w500:string)
            n260 = String Subset(string=w503, offset (0)=7, length (rest)=1 ("length (rest)")) -> (substring=w501:string)
            n261 = Decimal String To Number(string=w487) -> (number=w488:i32)  [unwired: 2 in, 1 out]
            n262 = Decimal String To Number(string=w492) -> (number=w491:i32)  [unwired: 2 in, 1 out]
            n263 = Decimal String To Number(string=w493) -> (number=w494:i32)  [unwired: 2 in, 1 out]
            n264 = Decimal String To Number(string=w496) -> (number=w495:i32)  [unwired: 2 in, 1 out]
            n265 = Decimal String To Number(string=w497) -> (number=w498:i32)  [unwired: 2 in, 1 out]
            n266 = Decimal String To Number(string=w500) -> (number=w499:i32)  [unwired: 2 in, 1 out]
            n267 = Decimal String To Number(string=w501) -> (number=w502:i32)  [unwired: 2 in, 1 out]
            n268 = Not Equal To 0?(x=w488) -> (x != 0?=w485:bool)
            n269 = Not Equal To 0?(x=w491) -> (x != 0?=w454:bool)
            n270 = Not Equal To 0?(x=w494) -> (x != 0?=w453:bool)
            n271 = Not Equal To 0?(x=w495) -> (x != 0?=w484:bool)
            n272 = Not Equal To 0?(x=w498) -> (x != 0?=w483:bool)
            n273 = Not Equal To 0?(x=w499) -> (x != 0?=w452:bool)
            n274 = Not Equal To 0?(x=w502) -> (x != 0?=w482:bool)
            n275 = call "ViscometerZeroFGV.vi"("Enum"=enum16{"Set RPM", "Set Zero", "Get Value"}."Get Value") -> ("RPM_read"=→"final_RPM":dbl)  [unwired: 13 in, 1 out]
            n276 = local write "Invalid Command Received"(w485) -> ()
            n277 = local write "Diagnostics Error"(w454) -> ()
            n278 = local write "Motor Circuit Error"(w453) -> ()
            n279 = local write "Auto-zero Complete"(w484) -> ()
            n280 = local write "Motor Stopped"(w483) -> ()
            n281 = local write "Motor On"(w452) -> ()
            n282 = local write "Control Circuitry Enabled"(w482) -> ()
            n283 = Build Array(w454, w453, w452) -> (w459:bool[])
            n284 = Or Array Elements(Boolean array=w459) -> (logical OR=w458:bool)
            n285 = Select(t=Brookfield_type-def."Error", s=w458, f=Brookfield_type-def."Disconnect") -> (s? t:f=w455:T1)
            n286 = Wait (ms)(milliseconds to wait=u32 500) -> ()  [unwired: 1 out]
          }
          frame "Error" {
            n287 = case shown="\"Set Speed\"" w510 {
              tunnel: [Brookfield_type-def."Disconnect" Brookfield_type-def."Disconnect" Brookfield_type-def."Stop Motor" Brookfield_type-def."Disconnect" Brookfield_type-def."Stop Motor" Brookfield_type-def."Stop Motor" Brookfield_type-def."Disconnect"] -> w513
              frame "Initialize", Default {
              }
              frame "Enable" {
              }
              frame "Ready" {
              }
              frame "Zero" {
              }
              frame "Set Speed" {
              }
              frame "Read" {
              }
              frame "Stop Motor" {
              }
            }
          }
          frame "Disconnect" {
            n288 = flat-sequence {
              tunnel: w525 -> [w528]
              tunnel: w524 -> [w527]
              tunnel: [TRUE] -> w523
              frame #0 {
                n289 = Get Date/Time In Seconds() -> (seconds since 1Jan1904=→"end_time":timestamp)
                n290 = VISA Close(VISA resource name=w528, error in (no error)=w527) -> ()  [unwired: 1 out]
              }
              frame #1 {
                n291 = local read "start_time"() -> (w530:timestamp)
                n292 = local read "end_time"() -> (w531:timestamp)
                n293 = Subtract(x=w531, y=w530) -> (x-y=→"ET (s)":dbl)
              }
            }
          }
        }
        n294 = Wait (ms)(milliseconds to wait=u32 100) -> ()  [unwired: 1 out]
        "Enum" <- w10
        "error out" <- w19
      }
      "TorqueArray" <- w3
      "TempArray" <- w6
      "Loop Tracker" <- w4
      n295 = call <vilib>:"Std Deviation and Variance.vi"("X"=w3) -> ("mean"=→"tau_mean":dbl, "standard deviation"=→"tau_std":dbl)  [unwired: 1 in, 1 out]
      "ReconnectAttempts" <- 0
    }
    frame #1 {
      n296 = local read "LogData? (T)"() -> (w533:bool)
      n297 = case shown="True" w533 {
        frame False {
        }
        frame True {
          w538 = "\r\n"
          w539 = "," ("delimiter (Tab)")
          w540 = "%.5f" ("format (%.3f)")
          n298 = local read "TorqueArray"() -> (w535:dbl[])
          n299 = local read "TempArray"() -> (w536:dbl[])
          n300 = local read "Zero_read"() -> (w534:dbl)
          n301 = Array To Spreadsheet String(delimiter (Tab)=w539, array=w535, 3:w540) -> (spreadsheet string=w544:string)
          n302 = Array To Spreadsheet String(delimiter (Tab)=w539, array=w536, 3:w540) -> (spreadsheet string=w543:string)
          n303 = Format Into String(format string=w540, w534) -> (resulting string=w542:string)  [unwired: 2 in, 1 out]
          n304 = Concatenate Strings("C:\\Users\\MUSE_V2\\Desktop\\Viscosity\\", "GUID", ".txt" ("string")) -> (w549:string)
          n305 = Concatenate Strings(w544, w538, w543, w538, w542, w538, "***" ("string")) -> (w541:string)
          "log_string" <- w541
          n306 = String To Path(string=w549) -> (path=w547:path)
          n307 = Open/Create/Replace File(file path (use dialog)=w547, operation (0:open)=T2."open or create") -> (refnum out=w548:refnum<file>)  [unwired: 4 in, 2 out]
          n308 = Write to Text File(file (use dialog)=w548, text=w541) -> ()  [unwired: 2 in, 3 out]
        }
      }
    }
  }
